vi "STFT_Freq2Mel_Mapper.vi"(8 "df":sgl, 11 "spectral map":sgl[][](array[numeric])) -> (3 "spectral map out":sgl[][](array[numeric]))   [LabVIEW 2020]
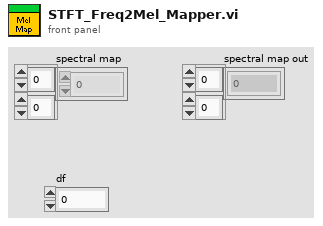
[diagram p1: front panel]
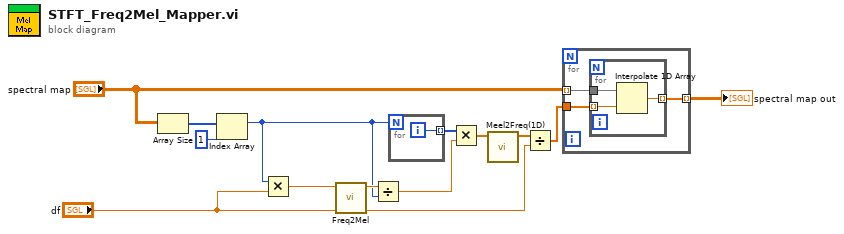
[diagram p0: block diagram]
diagram:
  n1 = Array Size(array="spectral map") -> (size(s)=w12:i32[])
  n2 = Index Array(array=w12, index=1) -> (element=w2:i32)
  n3 = Multiply(x=w2, y="df") -> (x*y=w13:sgl)
  n4 = call "Freq2Mel.vi"("F"=w13) -> ("Mel"=w9:dbl)  [unwired: 10 in]
  n5 = Divide(x=w9, y=w2) -> (x/y=w10:dbl)
  n6 = for {
    N: w2 -> [_]
    tunnel: [w14] -> w6 mode=indexing
    i -> [w14]
  }
  n7 = Multiply(x=w6, y=w10) -> (x*y=w7:dbl[])
  n8 = call "Meel2Freq(1D).vi"("Mel"=w7) -> ("Freq"=w8:dbl[])  [unwired: 10 in]
  n9 = Divide(x=w8, y="df") -> (x/y=w11:dbl[])
  n10 = for {
    tunnel: "spectral map" -> [w17] mode=indexing
    tunnel: [w16] -> w5 mode=indexing
    tunnel: w11 -> [w15]
    n11 = for {
      tunnel: w17 -> [w19]
      tunnel: w15 -> [w20] mode=indexing
      tunnel: [w18] -> w16 mode=indexing
      n12 = Interpolate 1D Array(1:w20, 2:w19) -> (0:w18:sgl)
    }
  }
  "spectral map out" <- w5
